vi "Cal Inst Main.vi"(10 "Master":refnum<queue>, 11 "Stand Alone?":bool=TRUE) -> ()   [LabVIEW 2013, in "Cal Inst.lvlib"]
doc: "This Continuous Measurement sample project is based on the Queued Message Handler template.\n\nThe Event Handling Loop generates messages based on user interface actions.\n\nThe Message Handling Loop processes messages generated by the Event Handling Loop, or by other messages. There are also Acquisition and Logging message handling loop subVIs, and a chart updating loop."
uses:
  Cal Inst.lvlib
  controls/electrical2.ctl
  support/Message Queue/Message Cluster.ctl
  Settings/Settings.ctl
  Acquisition/Hardware Configuration.ctl
  Logging/Logging Configuration.ctl
  controls/Cal Inst UI Data.ctl
  controls/Cal Inst UI State.ctl
  <vilib>/Utility/error.llb/Error Cluster From Error Code.vi
  <vilib>/ErrorRing/Error Ring.xnode
  Acquisition/Cal Inst Acquisition.lvlib
  Logging/Cal Inst Logging.lvlib
  Settings/Cal Inst Settings.lvlib
  support/User Event - Stop/Cal Inst User Event - Stop.lvlib
  support/Message Queue/Cal Inst Message Queue.lvlib
panel:
  in  "Base Path":path=path "C:/Users/dhstuart/Dropbox/CLTC/CaliforniaInstrumentsIxSeries"
  out "Electrical Data":T1
  in  "Power \nToggle":bool
  in  "Save Data":bool
  in  "Settings":bool
  in  "Start Acquisition":bool
  in  "Stop":bool
  in  "Exit":bool
  out "Status":string
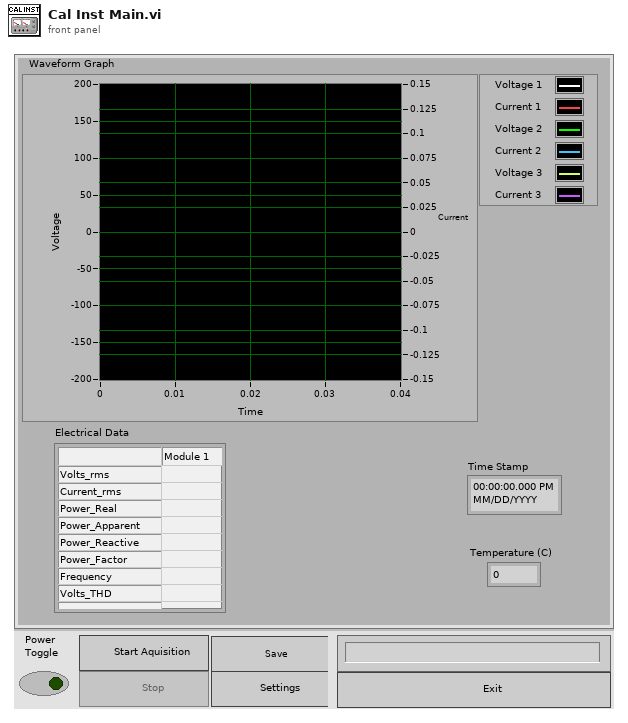
[diagram p1: front panel]
types:
  T1 = typedef "Cal Inst.lvlib/Cal Inst Acquisition.lvlib/electrical2.ctl" = cluster{"Time Stamp":timestamp, "Temperature (C)":dbl, "Electrical Data":string[][], "Waveform Graph":waveform(dbl)[]}
  T2 = typedef "Cal Inst.lvlib/Cal Inst UI State.ctl" = enum16{"Idle", "Acquiring and Logging", "Waiting for Exit", "Waiting for Exit (Acq Stopped)", "Waiting for Exit (Log Stopped)", "Waiting for Stop", "Waiting for Stop (Acq Stopped)", "Waiting for Stop (Log Stopped)"}
  T3 = typedef "Cal Inst.lvlib/Cal Inst UI Data.ctl" = cluster{"Start Ref":refnum<vi>, "Stop Ref":refnum<vi>, "Settings Ref":refnum<vi>, "Exit Ref":refnum<vi>, "Status Ref":refnum<vi>, "Electrical Data Ref":refnum<vi>, "Save Ref":refnum<vi>, "Connect to Instrument":refnum<vi>}
  T4 = typedef "Cal Inst.lvlib/Cal Inst Settings.lvlib/Settings.ctl" = cluster{"Hardware Configuration":T5, "Logging Configuration":T6}
  T5 = typedef "Cal Inst.lvlib/Cal Inst Acquisition.lvlib/Hardware Configuration.ctl" = cluster{"VISA Refnum in":refnum<visa-resource-name>, "Serial Configuration":cluster{"Baud Rate":u32, "Flow Control":u16}, "Voltage Level (0V)":dbl, "Output Phase(s) (1-Phase)":u16, "Active Phase (1:Phase 1)":i32, "Naked Sphere Phase":i32, "Insulated Sphere Phase":i32}
  T6 = typedef "Cal Inst.lvlib/Cal Inst Logging.lvlib/Logging Configuration.ctl" = cluster{"Log File Base Path":path, "TDMS File Reference":refnum<k34>}
  T7 = typedef "Cal Inst.lvlib/Cal Inst Message Queue.lvlib/All Message Queues.ctl" = cluster{"Master":refnum<queue>, "UI":refnum<queue>, "Acquisition":refnum<queue>, "Logging":refnum<queue>}
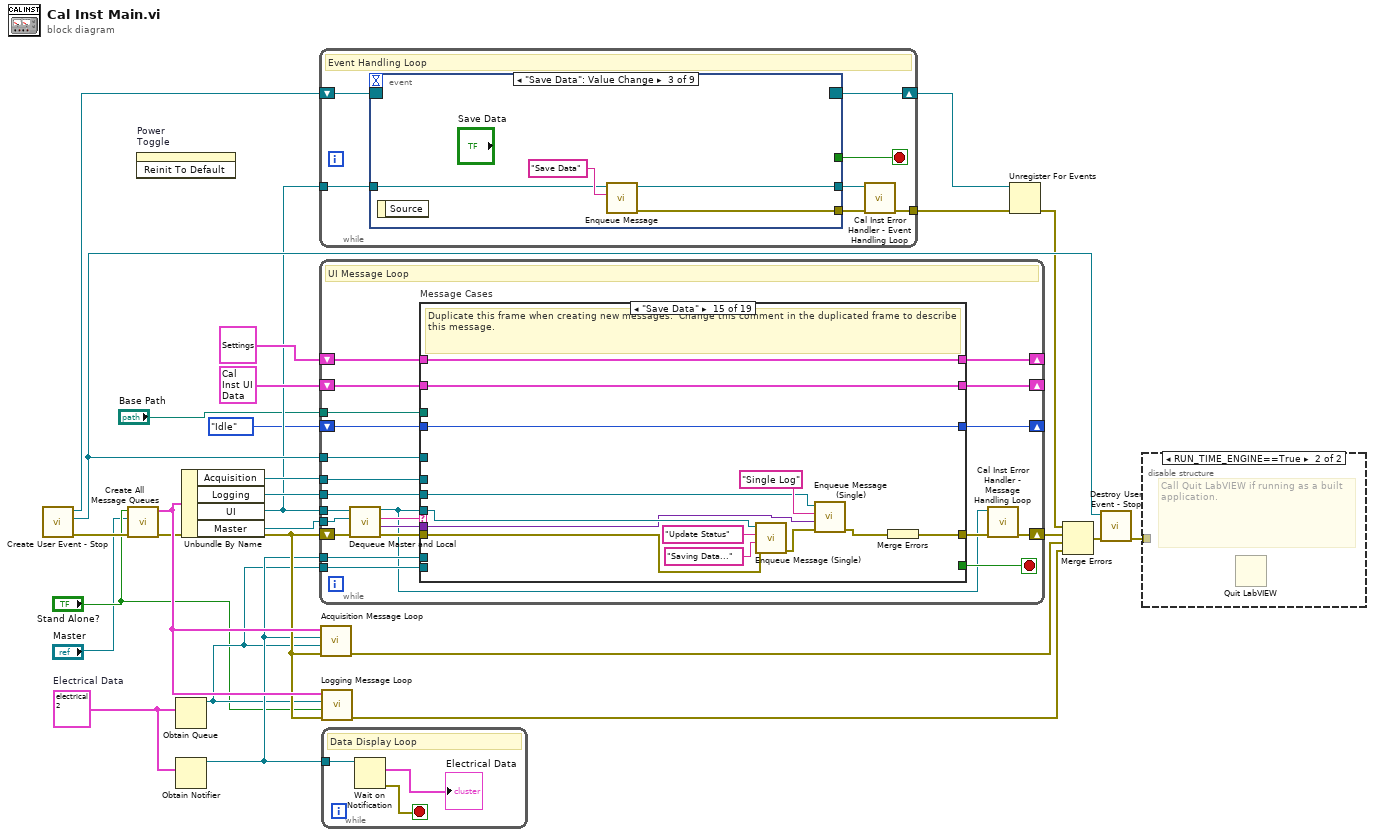
[diagram p0: block diagram]
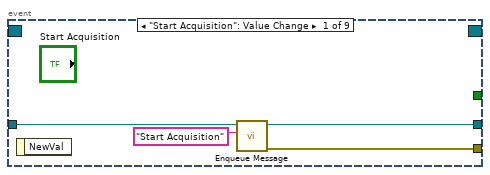
[diagram p3: hidden frame]
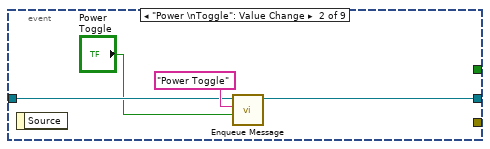
[diagram p4: hidden frame]
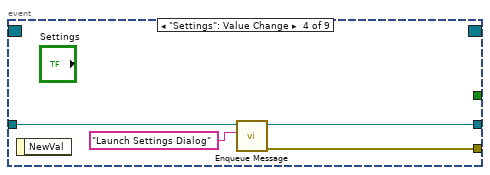
[diagram p5: hidden frame]
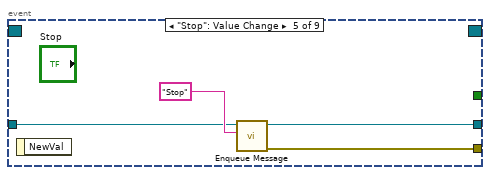
[diagram p6: hidden frame]
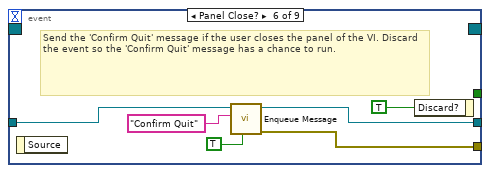
[diagram p7: hidden frame]
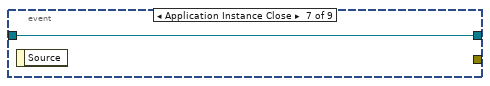
[diagram p8: hidden frame]
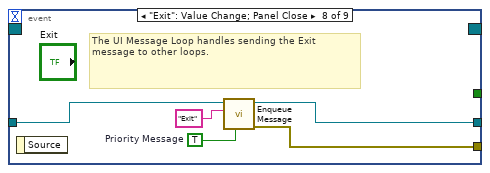
[diagram p9: hidden frame]
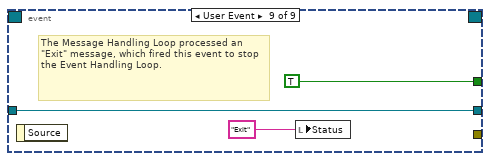
[diagram p10: hidden frame]
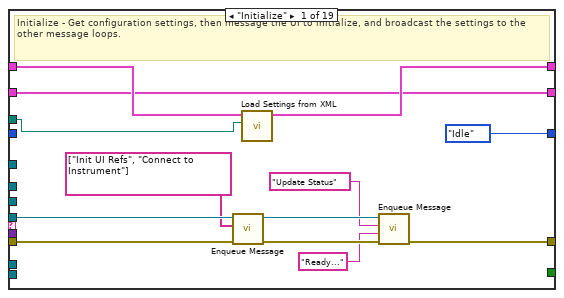
[diagram p11: hidden frame]
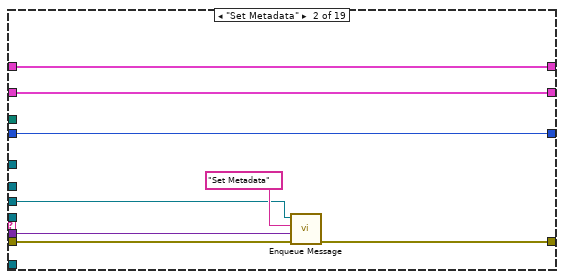
[diagram p12: hidden frame]
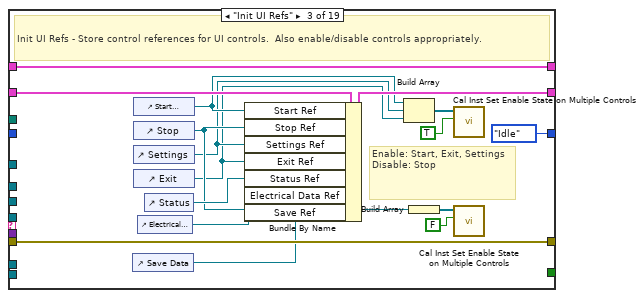
[diagram p13: hidden frame]
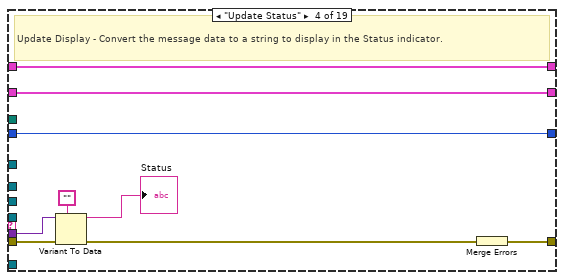
[diagram p14: hidden frame]
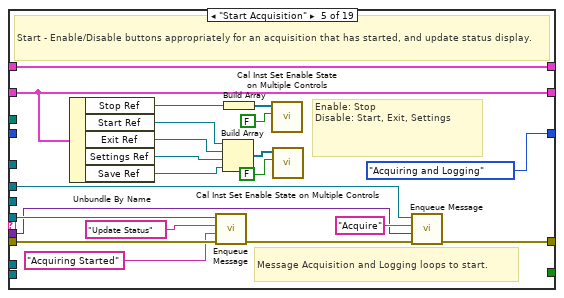
[diagram p15: hidden frame]
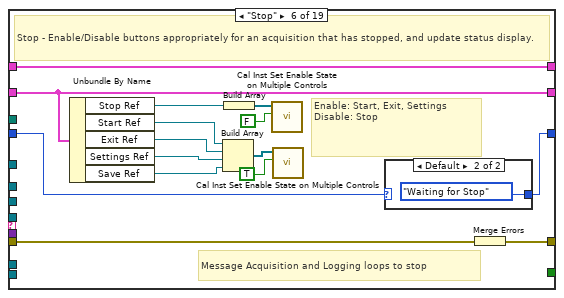
[diagram p16: hidden frame]
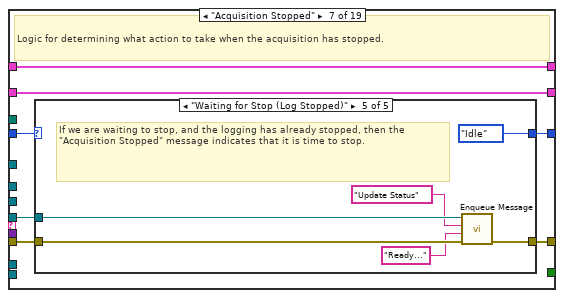
[diagram p18: hidden frame]
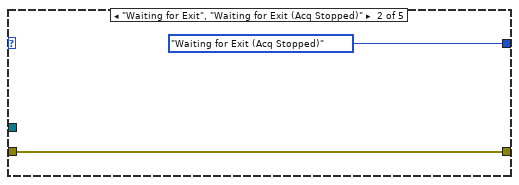
[diagram p20: hidden frame]
diagram:
  w7 = T1 {"Time Stamp"=timestamp(0 s since 1904-01-01), "Temperature (C)"=0.0, "Electrical Data"=[], "Waveform Graph"=[]}  # Electrical Data
  n1 = call "Create User Event - Stop.vi"() -> ("error out"=w21:errorcluster, "User Event - Stop"=w23:refnum<user-event>, "Stop Event Registration Refnum"=w24:refnum<event-registration>)  [unwired: 9 in]
  n2 = call "Create All Message Queues.vi"("error in (no error)"=w21, "Master Queue In"="Master", "Stand alone?"="Stand Alone?") -> ("error out"=w18:errorcluster, "Message Queues out"=w20:T7)  [unwired: 7 in]
  n3 = invoke on="Power \nToggle" class="Bool (strict)" method="Reinit To Default"() -> ()  [unwired: 3 in, 3 out]
  n4 = Obtain Queue(element data type=w7) -> (queue out=w5:refnum<queue>)  [unwired: 4 in, 2 out]
  n5 = Obtain Notifier(notification data type=w7) -> (notifier out=w6:refnum<notifier>)  [unwired: 3 in, 2 out]
  n6 = Unbundle By Name(w20) -> ("Acquisition"=w13:refnum<queue>, "Logging"=w12:refnum<queue>, "UI"=w11:refnum<queue>, "Master"=w2:refnum<queue>)
  n7 = while {
    tunnel: w11 -> [w32]
    tunnel: [w29] -> w25
    shift-right: [w31] -> w15
    shift-left: w24 -> [w33]
    stop <- w30 stop-if-true
    # "Event Handling Loop"
    n8 = event shown="[2] \"Save Data\": Value Change" {
      selector: w33 -> [_ _ _ _ _ _ _ _ _]
      dyn-events: [_ _ _ _ _ _ _ _ _] -> w31
      timeout: _ -> [_ _ _ _ _ _ _ _ _]
      tunnel: [_ _ _ _ _ _ _ _ TRUE ("Discard?")] -> w30
      tunnel: w32 -> [w37 w40 w42 w47 w52 w57 w60 w62 w66]
      tunnel: [w35 _ w43 w49 w51 w55 _ w65 _] -> w28
      tunnel: [w34 w39 w44 w46 w50 w56 w60 w61 w66] -> w27
      event "Start Acquisition": Value Change {
        n9 = event-data() -> ()  [unwired: 1 in, 1 out]
        n10 = call-poly "Enqueue Message.vi"("Message"="Start Acquisition", "Message Queue"=w37) -> ("error out"=w35:errorcluster, "dup Message Queue"=w34:refnum<queue>)  [unwired: 8 in]
      }
      event "Power \nToggle": Value Change {
        n11 = event-data() -> ()  [unwired: 1 in, 1 out]
        n12 = call-poly "Enqueue Message.vi"("Message Data"="Power \nToggle", "Message"="Power Toggle", "Message Queue"=w40) -> ("dup Message Queue"=w39:refnum<queue>)  [unwired: 7 in, 1 out]
      }
      event "Save Data": Value Change {
        n13 = event-data() -> ()  [unwired: 1 in, 1 out]
        n14 = call-poly "Enqueue Message.vi"("Message"="Save Data", "Message Queue"=w42) -> ("error out"=w43:errorcluster, "dup Message Queue"=w44:refnum<queue>)  [unwired: 8 in]
      }
      event "Settings": Value Change {
        n15 = event-data() -> ()  [unwired: 1 in, 1 out]
        n16 = call-poly "Enqueue Message.vi"("Message"="Launch Settings Dialog", "Message Queue"=w47) -> ("error out"=w49:errorcluster, "dup Message Queue"=w46:refnum<queue>)  [unwired: 8 in]
      }
      event "Stop": Value Change {
        n17 = event-data() -> ()  [unwired: 1 in, 1 out]
        n18 = call-poly "Enqueue Message.vi"("Message"="Stop", "Message Queue"=w52) -> ("error out"=w51:errorcluster, "dup Message Queue"=w50:refnum<queue>)  [unwired: 8 in]
      }
      event Panel Close? {
        # "Send the 'Confirm Quit' message if the user closes the panel of the VI. Discard the event so the 'Confirm Quit' message has a chance to run."
        n19 = event-data() -> ()  [unwired: 1 in, 1 out]
        n20 = call-poly "Enqueue Message.vi"("Priority Message? (F)"=TRUE, "Message"="Confirm Quit", "Message Queue"=w57) -> ("error out"=w55:errorcluster, "dup Message Queue"=w56:refnum<queue>)  [unwired: 7 in]
        n21 = event-data("Discard?"=TRUE) -> ()  [unwired: 1 in, 1 out]
      }
      event Application Instance Close {
        n22 = event-data() -> ()  [unwired: 1 in, 1 out]
      }
      event "Exit": Value Change; Panel Close {
        w63 = TRUE  # Priority Message
        # "The UI Message Loop handles sending the Exit message to other loops."
        n23 = event-data() -> ()  [unwired: 1 in, 1 out]
        n24 = call-poly "Enqueue Message.vi"("Priority Message? (F)"=w63, "Message"="Exit", "Message Queue"=w62) -> ("error out"=w65:errorcluster, "dup Message Queue"=w61:refnum<queue>)  [unwired: 7 in]
      }
      event User Event {
        # "The Message Handling Loop processed an \"Exit\" message, which fired this event to stop the Event Handling Loop."
        n25 = event-data() -> ()  [unwired: 1 in, 1 out]
        n26 = local write "Status"("Exit" ("Exit String")) -> ()
      }
    }
    n27 = call "Cal Inst Error Handler - Event Handling Loop.vi"("error in (no error)"=w28, "Message Queue"=w27) -> ("dup error in"=w29:errorcluster)  [unwired: 8 in, 1 out]
  }
  n28 = while {
    tunnel: w11 -> [w74]
    tunnel: w23 -> [w89]
    shift-right: [w82] -> w26
    shift-left: w18 -> [w76]
    shift-right: [w88] -> _
    shift-left: T4 {"Hardware Configuration"={"VISA Refnum in"="", "Serial Configuration"={"Baud Rate"=0, "Flow Control"=0}, "Voltage Level (0V)"=0.0, "Output Phase(s) (1-Phase)"=0, "Active Phase (1:Phase 1)"=0, "Naked Sphere Phase"=0, "Insulated Sphere Phase"=0}, "Logging Configuration"={"Log File Base Path"=path "", "TDMS File Reference"=refnum}} ("Settings") -> [w87]
    shift-right: [w85] -> _
    shift-left: T3 {"Start Ref"=refnum, "Stop Ref"=refnum, "Settings Ref"=refnum, "Exit Ref"=refnum, "Status Ref"=refnum, "Electrical Data Ref"=refnum, "Save Ref"=refnum, "Connect to Instrument"=refnum} ("Measurement UI Controls") -> [w86]
    tunnel: w13 -> [w84]
    tunnel: w12 -> [w83]
    shift-right: [w79] -> _
    shift-left: Cal_Inst_UI_State."Idle" ("UI State") -> [w80]
    tunnel: w6 -> [w78]
    tunnel: w5 -> [w77]
    tunnel: w2 -> [w73]
    tunnel: "Base Path" -> [w69]
    stop <- w90 stop-if-true
    # "UI Message Loop"
    n29 = call "Dequeue Master and Local.vi"("error in (no error)"=w76, "Master Queue In"=w73, "UI In"=w74) -> ("error out"=w75:errorcluster, "Message Data"=w72:variant, "Message"=w71:string, "UI Out"=w70:refnum<queue>)  [unwired: 5 in]
    n30 = case "Message Cases" shown="\"Save Data\"" w71 {
      selector: w71 -> [_ _ _ _ _ _ _ _ _ _ _ _ _ _ _ _ _ w348 _]
      tunnel: w70 -> [w95 _ _ _ w157 _ w177 w202 _ w242 w256 w267 w301 _ w324 _ _ _ _]
      tunnel: w75 -> [w94 w109 w127 w135 w156 w158 w178 w203 w230 w244 w259 w266 w308 w315 w321 w330 w341 _ w359]
      tunnel: [w99 w108 w127 w136 w143 w172 w175 w200 w236 w239 w255 w265 w309 w314 w328 w337 w346 w347 w359] -> w81
      tunnel: [_ _ _ _ _ _ _ _ _ _ _ _ TRUE _ _ _ _ _ _] -> w90
      tunnel: w72 -> [_ w107 _ w134 w137 _ _ _ _ _ w257 _ _ _ w316 w331 _ _ _]
      tunnel: w89 -> [_ _ _ _ _ _ _ _ _ _ _ _ w307 _ _ _ _ _ _]
      tunnel: [w102 w111 w126 w130 w155 w171 w181 w206 w234 w241 w263 w270 w305 w313 w327 w334 w339 w351 w362] -> w88
      tunnel: w87 -> [w103 w111 w126 w130 w155 w171 w181 w206 w234 w245 w263 w270 w305 w313 w327 w334 w339 w351 w362]
      tunnel: w86 -> [w96 w110 w125 w129 w152 w170 w180 w205 w228 w238 w262 w269 w303 w312 w326 w336 w345 w350 w361]
      tunnel: [w96 w110 w123 w129 w152 w170 w180 w205 w228 w238 w262 w269 w303 w312 w326 w336 w345 w350 w361] -> w85
      tunnel: w84 -> [_ _ _ _ w142 _ _ _ w227 _ _ _ w294 _ _ w332 w342 _ _]
      tunnel: w83 -> [_ w105 _ _ _ _ _ _ w226 _ _ _ w302 _ w317 _ _ _ _]
      tunnel: w80 -> [_ w104 _ w128 _ w160 w179 w204 w225 w237 w251 w268 _ w311 w325 w335 w344 w349 w360]
      tunnel: [Cal_Inst_UI_State."Idle" ("UI State") w104 Cal_Inst_UI_State."Idle" ("UI State") w128 Cal_Inst_UI_State."Acquiring and Logging" ("UI State") w161 w176 w201 w225 w237 w251 w264 Cal_Inst_UI_State."Idle" ("UI State") w311 w325 w335 w344 w349 w360] -> w79
      tunnel: w78 -> [_ _ _ _ _ _ _ _ _ _ _ _ w296 _ _ _ _ _ _]
      tunnel: w77 -> [_ _ _ _ _ _ _ _ _ _ _ _ w295 _ _ _ _ _ _]
      tunnel: w69 -> [w91 _ _ _ _ _ _ _ _ _ _ _ _ _ _ _ _ _ _]
      frame "Initialize" {
        # "Initialize - Get configuration settings, then message the UI to initialize, and broadcast the settings to the other message loops."
        n31 = call-poly "Enqueue Message.vi"("error in (no error)"=w94, "Message Array"=string[] ["Init UI Refs", "Connect to Instrument"], "Message Queue"=w95) -> ("error out"=w101:errorcluster, "dup Message Queue"=w100:refnum<queue>)  [unwired: 7 in]
        n32 = call "Load Settings from XML.vi"("Base Path"=w91, "Settings in"=w103) -> ("Settings out"=w102:T4)  [unwired: 8 in, 1 out]
        n33 = call-poly "Enqueue Message.vi"("error in (no error)"=w101, "Message Data"="Ready..." ("Ready..."), "Message"="Update Status", "Message Queue"=w100) -> ("error out"=w99:errorcluster)  [unwired: 6 in, 1 out]
      }
      frame "Set Metadata" {
        n34 = call-poly "Enqueue Message.vi"("error in (no error)"=w109, "Message Data"=w107, "Message"="Set Metadata", "Message Queue"=w105) -> ("error out"=w108:errorcluster)  [unwired: 6 in, 1 out]
      }
      frame "Init UI Refs" {
        # "Enable: Start, Exit, Settings\nDisable: Stop"
        # "Init UI Refs - Store control references for UI controls.  Also enable/disable controls appropriately."
        n35 = control-ref of="Save Data"() -> (w112:refnum<vi>)
        n36 = control-ref of="Start Acquisition"() -> (w117:refnum<vi>)
        n37 = control-ref of="Stop"() -> (w118:refnum<vi>)
        n38 = control-ref of="Settings"() -> (w116:refnum<vi>)
        n39 = control-ref of="Exit"() -> (w115:refnum<vi>)
        n40 = control-ref of="Electrical Data"() -> (w113:refnum<vi>)
        n41 = control-ref of="Status"() -> (w124:refnum<vi>)
        n42 = Bundle By Name(cluster=w125, "Start Ref"=w117, "Stop Ref"=w118, "Settings Ref"=w116, "Exit Ref"=w115, "Status Ref"=w124, "Electrical Data Ref"=w113, "Save Ref"=w112) -> (w123:T3)
        n43 = Build Array(w117, w116, w115) -> (w121:refnum<vi>[])
        n44 = Build Array(w118) -> (w120:refnum<vi>[])
        n45 = call "Cal Inst Set Enable State on Multiple Controls.vi"("Enable?"=TRUE, "Controls"=w121) -> ()  [unwired: 10 in]
        n46 = call "Cal Inst Set Enable State on Multiple Controls.vi"("Enable?"=FALSE, "Controls"=w120) -> ()  [unwired: 10 in]
      }
      frame "Update Status" {
        # "Update Display - Convert the message data to a string to display in the Status indicator."
        n47 = Variant To Data(error in=w135, type="", Variant=w134) -> (data=→"Status":string, error out=w132:errorcluster)
        n48 = Merge Errors(w132) -> (w136:errorcluster)
      }
      frame "Start Acquisition" {
        # "Message Acquisition and Logging loops to start."
        # "Enable: Stop\nDisable: Start, Exit, Settings"
        # "Start - Enable/Disable buttons appropriately for an acquisition that has started, and update status display."
        n49 = Unbundle By Name(w152) -> ("Stop Ref"=w147:refnum<vi>, "Start Ref"=w146:refnum<vi>, "Exit Ref"=w145:refnum<vi>, "Settings Ref"=w144:refnum<vi>, "Save Ref"=w139:refnum<vi>)
        n50 = call-poly "Enqueue Message.vi"("error in (no error)"=w156, "Message Data"="Acquiring Started" ("Acquiring and Logging..."), "Message"="Update Status", "Message Queue"=w157) -> ("error out"=w138:errorcluster)  [unwired: 6 in, 1 out]
        n51 = Build Array(w146, w145, w144, w139) -> (w150:refnum<vi>[])
        n52 = Build Array(w147) -> (w149:refnum<vi>[])
        n53 = call "Cal Inst Set Enable State on Multiple Controls.vi"("Enable?"=FALSE, "Controls"=w149) -> ()  [unwired: 10 in]
        n54 = call "Cal Inst Set Enable State on Multiple Controls.vi"("Enable?"=FALSE, "Controls"=w150) -> ()  [unwired: 10 in]
        n55 = call-poly "Enqueue Message.vi"("error in (no error)"=w138, "Message Data"=w137, "Message"="Acquire", "Message Queue"=w142) -> ("error out"=w143:errorcluster)  [unwired: 6 in, 1 out]
      }
      frame "Stop" {
        # "Message Acquisition and Logging loops to stop"
        # "Enable: Start, Exit, Settings\nDisable: Stop"
        # "Stop - Enable/Disable buttons appropriately for an acquisition that has stopped, and update status display."
        n56 = Unbundle By Name(w170) -> ("Stop Ref"=w165:refnum<vi>, "Start Ref"=w164:refnum<vi>, "Exit Ref"=w163:refnum<vi>, "Settings Ref"=w162:refnum<vi>, "Save Ref"=w159:refnum<vi>)
        n57 = Build Array(w164, w163, w162, w159) -> (w168:refnum<vi>[])
        n58 = Build Array(w165) -> (w167:refnum<vi>[])
        n59 = call "Cal Inst Set Enable State on Multiple Controls.vi"("Enable?"=FALSE, "Controls"=w167) -> ()  [unwired: 10 in]
        n60 = call "Cal Inst Set Enable State on Multiple Controls.vi"("Enable?"=TRUE, "Controls"=w168) -> ()  [unwired: 10 in]
        n61 = case shown="Default" w160 {
          selector: w160 -> [w173 _]
          tunnel: [w173 Cal_Inst_UI_State."Waiting for Stop" ("UI State")] -> w161
          frame "Waiting for Exit" {
          }
          frame Default {
          }
        }
        n62 = Merge Errors(w158) -> (w172:errorcluster)
      }
      frame "Acquisition Stopped" {
        # "Logic for determining what action to take when the acquisition has stopped."
        n63 = case shown="\"Waiting for Stop (Log Stopped)\"" w179 {
          selector: w179 -> [w183 _ _ _ _]
          tunnel: w178 -> [w182 w185 w187 w193 w199]
          tunnel: w177 -> [_ _ _ w191 w196]
          tunnel: [w183 Cal_Inst_UI_State."Waiting for Exit (Acq Stopped)" ("UI State") Cal_Inst_UI_State."Waiting for Stop (Acq Stopped)" ("UI State") Cal_Inst_UI_State."Idle" ("UI State") Cal_Inst_UI_State."Idle" ("UI State")] -> w176
          tunnel: [w182 w185 w187 w192 w197] -> w175
          frame Default {
          }
          frame "Waiting for Exit", "Waiting for Exit (Acq Stopped)" {
          }
          frame "Waiting for Stop", "Waiting for Stop (Acq Stopped)" {
          }
          frame "Waiting for Exit (Log Stopped)" {
            # "If we are waiting to exit, and the logging has already stopped, then the \"Acquisition Stopped\" message indicates that it is time to exit."
            n64 = call-poly "Enqueue Message.vi"("Priority Message? (F)"=TRUE, "error in (no error)"=w193, "Message"="Exit", "Message Queue"=w191) -> ("error out"=w192:errorcluster)  [unwired: 6 in, 1 out]
          }
          frame "Waiting for Stop (Log Stopped)" {
            # "If we are waiting to stop, and the logging has already stopped, then the \"Acquisition Stopped\" message indicates that it is time to stop."
            n65 = call-poly "Enqueue Message.vi"("error in (no error)"=w199, "Message Data"="Ready..." ("Ready..."), "Message"="Update Status", "Message Queue"=w196) -> ("error out"=w197:errorcluster)  [unwired: 6 in, 1 out]
          }
        }
      }
      frame "Logging Stopped" {
        # "Logic for determining what action to take when the logging has stopped."
        n66 = case shown="\"Waiting for Stop (Acq Stopped)\"" w204 {
          selector: w204 -> [w208 _ _ _ _]
          tunnel: w203 -> [w207 w210 w212 w218 w221]
          tunnel: w202 -> [_ _ _ w216 w220]
          tunnel: [w208 Cal_Inst_UI_State."Waiting for Exit (Log Stopped)" ("UI State") Cal_Inst_UI_State."Waiting for Stop (Log Stopped)" ("UI State") Cal_Inst_UI_State."Idle" ("UI State") Cal_Inst_UI_State."Idle" ("UI State")] -> w201
          tunnel: [w207 w210 w212 w217 w219] -> w200
          frame Default {
          }
          frame "Waiting for Exit", "Waiting for Exit (Log Stopped)" {
          }
          frame "Waiting for Stop", "Waiting for Stop (Log Stopped)" {
          }
          frame "Waiting for Exit (Acq Stopped)" {
            # "If we are waiting to exit, and the acquisition has already stopped, then the \"Logging Stopped\" message indicates that it is time to exit."
            n67 = call-poly "Enqueue Message.vi"("Priority Message? (F)"=TRUE, "error in (no error)"=w218, "Message"="Exit", "Message Queue"=w216) -> ("error out"=w217:errorcluster)  [unwired: 6 in, 1 out]
          }
          frame "Waiting for Stop (Acq Stopped)" {
            # "If we are waiting to stop, and the acquisition has already stopped, then the \"Logging Stopped\" message indicates that it is time to stop."
            n68 = call-poly "Enqueue Message.vi"("error in (no error)"=w221, "Message Data"="Ready..." ("Ready..."), "Message"="Update Status", "Message Queue"=w220) -> ("error out"=w219:errorcluster)  [unwired: 6 in, 1 out]
          }
        }
      }
      frame "Broadcast settings" {
        w229 = "Update Settings" ("Message")
        # "Broadcast settings - Send the 'Update Settings' message to the Logging and Acquisition message loops."
        n69 = Unbundle By Name(w234) -> ("Hardware Configuration"=w233:T5, "Logging Configuration"=w232:T6)
        n70 = call-poly "Enqueue Message.vi"("Message Data"=w233, "Message"=w229, "Message Queue"=w227) -> ("error out"=w235:errorcluster)  [unwired: 7 in, 1 out]
        n71 = call-poly "Enqueue Message.vi"("error in (no error)"=w235, "Message Data"=w232, "Message"=w229, "Message Queue"=w226) -> ("error out"=w231:errorcluster)  [unwired: 6 in, 1 out]
        n72 = Merge Errors(w231, w230) -> (w236:errorcluster)
      }
      frame "Launch Settings Dialog" {
        # "Launch Settings Dialog - Launch the Settings Dialog when the user clicks the 'Settings' button."
        n73 = call "Settings Dialog.vi"("error in (no error)"=w244, "Settings in"=w245) -> ("error out"=w240:errorcluster, "Cancelled?"=w243:bool, "Settings out"=w241:T4)  [unwired: 6 in, 1 out]
        n74 = case shown="False" w243 {
          tunnel: w242 -> [w249 _]
          tunnel: w240 -> [w248 w250]
          tunnel: [w247 w250] -> w239
          frame False {
            n75 = call-poly "Enqueue Message.vi"("error in (no error)"=w248, "Message"="Broadcast Settings", "Message Queue"=w249) -> ("error out"=w247:errorcluster)  [unwired: 7 in, 1 out]
          }
          frame True {
          }
        }
      }
      frame "Error" {
        # "Error - Check the error message data and respond accordingly. This message is sent by the \"Error Handler\" VIs at the end of each loop in this application."
        n76 = Variant To Data(error in=w259, type=errorcluster {"status"=FALSE, "code"=0, "source"=""} ("error constant"), Variant=w257) -> (data=w261:errorcluster, error out=w258:errorcluster)
        n77 = call <vilib>:"Simple Error Handler.vi"("error in (no error)"=w261) -> ()  [unwired: 4 in, 5 out]
        n78 = call-poly "Enqueue Message.vi"("Priority Message? (F)"=TRUE, "Message"="Exit", "Message Queue"=w256) -> ("error out"=w254:errorcluster)  [unwired: 7 in, 1 out]
        n79 = Merge Errors(w254, w258) -> (w255:errorcluster)
      }
      frame "Confirm Quit" {
        # "Confirm Quit - Message that can confirm whether or not the user wants to exit the application."
        n80 = case shown="\"Acquiring and Logging\"" w268 {
          tunnel: w267 -> [w276 w280]
          tunnel: w266 -> [w275 w279]
          tunnel: [w274 w278] -> w265
          tunnel: [Cal_Inst_UI_State."Idle" ("UI State") w277] -> w264
          frame Default {
            # "If 'Confirm Quit' comes in while the system is idle, there is no need for a confirmation message."
            n81 = call-poly "Enqueue Message.vi"("Priority Message? (F)"=TRUE, "error in (no error)"=w275, "Message"="Exit", "Message Queue"=w276) -> ("error out"=w274:errorcluster)  [unwired: 6 in, 1 out]
          }
          frame "Acquiring and Logging" {
            n82 = Two Button Dialog(message="Are you sure you want to quit while the acquisition is running?" ("Confirm Quit Message"), 1:"No" ("No"), 2:"Yes" ("Yes")) -> (T button?=w281:bool)
            n83 = case shown="True" w281 {
              tunnel: w280 -> [_ w290]
              tunnel: w279 -> [w286 w291]
              tunnel: [w286 w289] -> w278
              tunnel: [Cal_Inst_UI_State."Acquiring and Logging" ("UI State") Cal_Inst_UI_State."Waiting for Exit" ("UI State")] -> w277
              frame False {
                # "User did not want to quit."
              }
              frame True {
                n84 = call-poly "Enqueue Message.vi"("error in (no error)"=w291, "Message"="Stop", "Message Queue"=w290) -> ("error out"=w289:errorcluster)  [unwired: 7 in, 1 out]
              }
            }
          }
        }
      }
      frame "Exit" {
        # "Don't check the error outs. The acquisition and logging queues may have already been released."
        # "Close references owned by the Main VI."
        # "Stop the VI"
        # "Exit - Fire the User Event to stop the Event Handling Loop.  Also send Exit messages to the Acquisition and Logging loops."
        n85 = Release Queue(queue=w301, error in (no error)=w308) -> (error out=w300:errorcluster)  [unwired: 1 in, 2 out]
        n86 = call "Fire User Event - Stop.vi"("User Event - Stop"=w307) -> ("error out"=w306:errorcluster)  [unwired: 10 in]
        n87 = Release Notifier(notifier=w296, error in (no error)=w300) -> (error out=w299:errorcluster)  [unwired: 1 in, 2 out]
        n88 = Release Queue(queue=w295, error in (no error)=w299) -> (error out=w298:errorcluster)  [unwired: 1 in, 2 out]
        n89 = call "Enqueue Message (Array).vi"("Message Data Array"=bool[] [FALSE, FALSE], "Message Array"=string[] ["Power Toggle", "Exit"], "Message Queue"=w294) -> ()  [unwired: 7 in, 2 out]
        n90 = call-poly "Enqueue Message.vi"("Message"="Exit", "Message Queue"=w302) -> ()  [unwired: 8 in, 2 out]
        n91 = Merge Errors(w306, w298) -> (w309:errorcluster)
      }
      frame "---Copy This Frame---" {
        # "Duplicate this frame when creating new messages.  Change this comment in the duplicated frame to describe this message."
        n92 = Merge Errors(w315) -> (w314:errorcluster)
      }
      frame "Save Data" {
        # "Duplicate this frame when creating new messages.  Change this comment in the duplicated frame to describe this message."
        n93 = call "Enqueue Message (Single).vi"("error in (no error)"=w321, "Message Data"="Saving Data..." ("Message"), "Message"="Update Status", "Message Queue"=w324) -> ("error out"=w320:errorcluster)  [unwired: 6 in, 1 out]
        n94 = call "Enqueue Message (Single).vi"("error in (no error)"=w320, "Message Data"=w316, "Message"="Single Log", "Message Queue"=w317) -> ("error out"=w319:errorcluster)  [unwired: 6 in, 1 out]
        n95 = Merge Errors(w319) -> (w328:errorcluster)
      }
      frame "Power Toggle" {
        # "Duplicate this frame when creating new messages.  Change this comment in the duplicated frame to describe this message."
        n96 = call-poly "Enqueue Message.vi"("error in (no error)"=w330, "Message Data"=w331, "Message"="Power Toggle", "Message Queue"=w332) -> ("error out"=w329:errorcluster)  [unwired: 6 in, 1 out]
        n97 = Merge Errors(w329) -> (w337:errorcluster)
      }
      frame "Connect to Instrument" {
        # "Duplicate this frame when creating new messages.  Change this comment in the duplicated frame to describe this message."
        n98 = Unbundle By Name(w339) -> ("Hardware Configuration"=w338:T5)
        n99 = call-poly "Enqueue Message.vi"("error in (no error)"=w341, "Message Data"=w338, "Message"="Start", "Message Queue"=w342) -> ("error out"=w340:errorcluster)  [unwired: 6 in, 1 out]
        n100 = Merge Errors(w340) -> (w346:errorcluster)
      }
      frame Default {
        # "'Default' case only runs if there is a message that isn't defined in any of the other cases.  Output a programming error."
        n101 = xnode "Error Ring"("parameter 0"=w348) -> ("error out"=w347:errorcluster)
      }
      frame "Ignore Message" {
        # "'Default' case only runs if there is a message that isn't defined in any of the other cases.  Output a programming error."
      }
    }
    n102 = call "Cal Inst Error Handler - Message Handling Loop.vi"("error in (no error)"=w81, "Message Queue"=w70) -> ("dup error in"=w82:errorcluster)  [unwired: 8 in, 1 out]
  }
  n103 = call "Acquisition Message Loop.vi"("error in (no error)"=w18, "Data Queue"=w5, "Data Notifier"=w6, "Message Queues"=w20) -> ("error out"=w22:errorcluster)  [unwired: 7 in]
  n104 = call "Logging Message Loop.vi"("error in (no error)"=w18, "Stand alone?"="Stand Alone?", "Data Queue"=w5, "Message Queues"=w20) -> ("error out"=w19:errorcluster)  [unwired: 7 in]
  n105 = while "Data Display Loop" {
    tunnel: w6 -> [w365]
    stop <- w364 stop-if-true
    # "Data Display Loop"
    n106 = Wait on Notification(notifier=w365) -> (notification=→"Electrical Data":T1, error out=w364:errorcluster)  [unwired: 3 in, 2 out]
  }
  n107 = Unregister For Events(event registration refnum=w15, error in=w25) -> (error out=w16:errorcluster)
  n108 = Merge Errors(w16, w26, w22, w19) -> (w8:errorcluster)
  n109 = call "Destroy User Event - Stop.vi"("error in (no error)"=w8, "User Event - Stop"=w23) -> ("error out"=w10:errorcluster)  [unwired: 9 in]
  n110 = disable-structure shown="RUN_TIME_ENGINE==True" {
    disable-tunnel: w10 -> [_ _]
    frame condition #0 (active) {
    }
    frame condition #1 {
      # "Call Quit LabVIEW if running as a built application."
      n111 = Quit LabVIEW() -> ()  [unwired: 1 in]
    }
  }
